vi "WM_CAP - Snap Window.vi"(7 "image data":T1) -> ()   [LabVIEW 2022 SP3]
uses:
  <vilib>/picture/picture.llb/imagedata.ctl
panel:
  out "Snap":picture
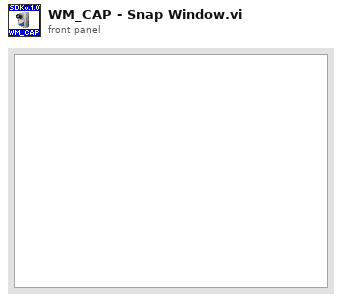
[diagram p1: front panel]
types:
  T1 = typedef "imagedata.ctl" = cluster{"image type":i32, "image depth":i32, "image":u8[], "mask":u8[], "colors":u32[], "Rectangle":cluster{"left":i16, "top":i16, "right":i16, "bottom":i16}}
  T2 = cluster{"left":i16, "top":i16, "right":i16, "bottom":i16}
  T3 = typedef "LVRectTypeDef.ctl" = cluster{"Left":i16, "Top":i16, "Right":i16, "Bottom":i16}
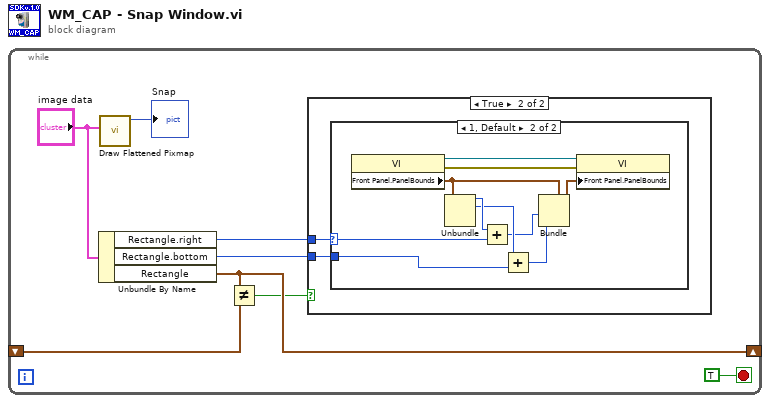
[diagram p0: block diagram]
diagram:
  n1 = while {
    shift-right: [w2] -> _
    shift-left: _ -> [w3]
    stop <- TRUE stop-if-true
    n2 = Unbundle By Name("image data") -> ("Rectangle.right"=w6:i16, "Rectangle.bottom"=w5:i16, "Rectangle"=w2:T2)
    n3 = call <vilib>:"Draw Flattened Pixmap.vi"("image data"="image data") -> ("new picture"=→"Snap":picture)  [unwired: 8 in]
    n4 = Not Equal?(x=w2, y=w3) -> (x != y?=w1:bool)
    n5 = case shown="True" w1 {
      tunnel: w6 -> [_ w10]
      tunnel: w5 -> [_ w9]
      frame False {
      }
      frame True {
        n6 = case shown="1, Default" w10 {
          selector: w10 -> [_ w15]
          tunnel: w9 -> [_ w13]
          frame 0 {
          }
          frame 1, Default {
            n7 = property class="VI"() -> (reference out=w19:refnum<vi>, error out=w18:errorcluster, "Front Panel.PanelBounds"=w17:T3)  [unwired: 2 in]
            n8 = Unbundle(w17) -> ("Left"=w16:i16, "Top"=w14:i16)  [unwired: 2 out]
            n9 = Add(x=w16, y=w15) -> (x+y=w12:i16)
            n10 = Add(x=w14, y=w13) -> (x+y=w11:i16)
            n11 = Bundle(cluster=w17, "Right"=w12, "Bottom"=w11) -> (w20:T3)  [unwired: 2 in]
            n12 = property class="VI"(reference=w19, error in=w18, "Front Panel.PanelBounds"=w20) -> ()  [unwired: 2 out]
          }
        }
      }
    }
  }
